vi "Visa Read-Write.vi"(8 "error in (no error)":errorcluster, 10 "Write buffer":string, 11 "VISA resource name":refnum<visa-resource-name>) -> (0 "error out":errorcluster, 2 "read buffer":string)   [LabVIEW 2018]
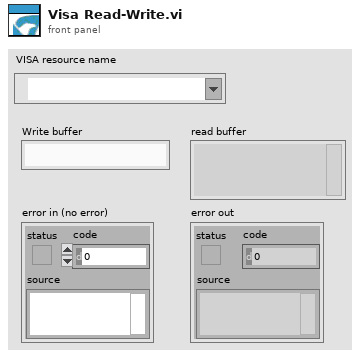
[diagram p1: front panel]
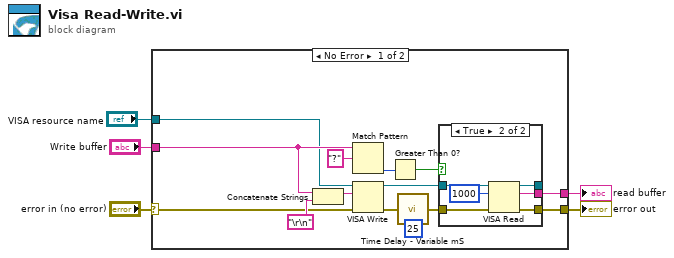
[diagram p0: block diagram]
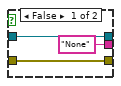
[diagram p2: hidden frame]
diagram:
  n1 = case shown="No Error" "error in (no error)" {
    selector: "error in (no error)" -> [w9 w29]
    tunnel: [w8 w29] -> w4
    tunnel: "Write buffer" -> [w10 _]
    tunnel: [w7 _] -> w2
    tunnel: "VISA resource name" -> [w6 _]
    frame No Error {
      n2 = Concatenate Strings(w10, "\r\n") -> (w15:string)
      n3 = Match Pattern(string=w10, regular expression="?") -> (offset past match=w18:i32)  [unwired: 1 in, 3 out]
      n4 = VISA Write(VISA resource name=w6, write buffer=w15, error in (no error)=w9) -> (VISA resource name out=w16:refnum<visa-resource-name>, error out=w13:errorcluster)  [unwired: 1 out]
      n5 = Greater Than 0?(x=w18) -> (x > 0?=w17:bool)
      n6 = call "Time Delay - Variable mS.vi"("milliseconds to wait"=u32 25, "error in (no error)"=w13) -> ("error out"=w12:errorcluster)  [unwired: 2 in]
      n7 = case shown="True" w17 {
        tunnel: w12 -> [w22 w28]
        tunnel: w16 -> [w21 w27]
        tunnel: [w22 w26] -> w8
        tunnel: ["None" ("read buffer") w24] -> w7
        tunnel: [w21 w23] -> _
        frame False {
        }
        frame True {
          n8 = VISA Read(VISA resource name=w27, byte count=u32 1000, error in (no error)=w28) -> (VISA resource name out=w23:refnum<visa-resource-name>, read buffer=w24:string, error out=w26:errorcluster)  [unwired: 1 out]
        }
      }
    }
    frame Error {
    }
  }
  "error out" <- w4
  "read buffer" <- w2
